vi "Read stop event.vi"(11 "GUI in":refnum<class "GUI.lvclass">) -> (1 "cmd event":refnum<user-event>, 2 "stop event":refnum<user-event>, 3 "GUI out":refnum<class "GUI.lvclass">)   [LabVIEW 2019, in "GUI.lvclass"]
uses:
  GUI.lvclass
  CmdData.ctl
  GUI.lvclass/GUI.ctl
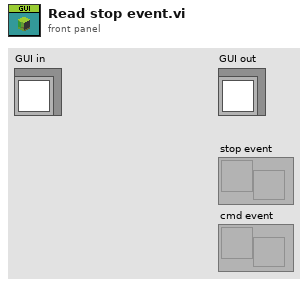
[diagram p1: front panel]
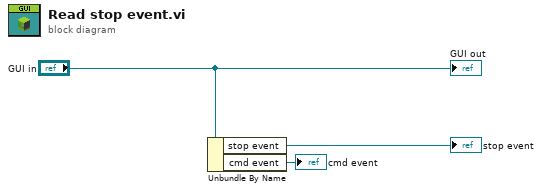
[diagram p0: block diagram]
diagram:
  n1 = Unbundle By Name("GUI in") -> ("stop event"=→"stop event":refnum<user-event>, "cmd event"=→"cmd event":refnum<user-event>)
  "GUI out" <- "GUI in"
